vi "Flatten Driver Parameters.vi"(4 "error in (no error)":errorcluster, 6 "Flattened Driver Parameters (\"\")":string, 7 "Driver Version":T1 {"Build Date/Time" format="%<%X\n%x>T"}) -> (0 "error out":errorcluster, 3 "Flattened Driver Parameters with Version":string)   [LabVIEW 2011]
uses:
  Summitek/Win32/Miscellaneous/OGAB Version.ctl
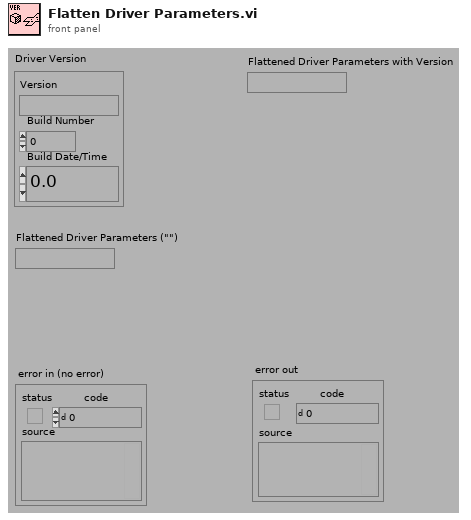
[diagram p1: front panel]
types:
  T1 = typedef "OGAB Version.ctl" = cluster{"Version":string, "Build Number":u32, "Build Date/Time":dbl}
  T2 = cluster{"Version":string, "Flattened Driver Parameters (\"\")":string}
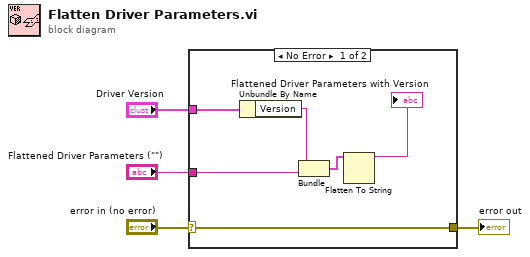
[diagram p0: block diagram]
diagram:
  n1 = case shown="No Error" "error in (no error)" {
    selector: "error in (no error)" -> [w8 w11]
    tunnel: [w8 w11] -> w3
    tunnel: "Flattened Driver Parameters (\"\")" -> [w7 _]
    tunnel: "Driver Version" -> [w6 _]
    frame No Error {
      n2 = Unbundle By Name(w6) -> ("Version"=w10:string)
      n3 = Bundle("Version"=w10, "Flattened Driver Parameters (\"\")"=w7) -> (w9:T2)  [unwired: 1 out]
      n4 = Flatten To String(anything=w9) -> (data string=→"Flattened Driver Parameters with Version":string)  [unwired: 1 in, 4 out]
    }
    frame Error {
    }
  }
  "error out" <- w3
